vi "Drive straight.vi"(8 "Start Time":dbl, 9 "Length(seconds)":dbl, 10 "Desired angle":dbl) -> (0 "Complete or not":bool, 2 "X Power":dbl)   [LabVIEW 2020]
uses:
  Robot Global Data.vi
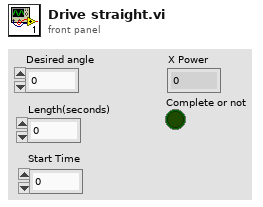
[diagram p1: front panel]
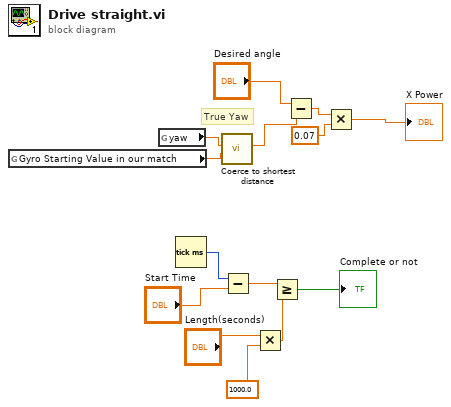
[diagram p0: block diagram]
diagram:
  # "True Yaw"
  n1 = global read "Robot Global Data.vi" "Gyro Starting Value in our match"() -> (w1:dbl)
  n2 = global read "Robot Global Data.vi" "yaw"() -> (w2:dbl)
  n3 = Tick Count (ms)() -> (millisecond timer value=w7:u32)
  n4 = call "Coerce to shortest distance.vi"("Angle 2"=w1, "Angle 1"=w2) -> ("Shortest distance"=w3:dbl)  [unwired: 9 in]
  n5 = Subtract(x=w7, y="Start Time") -> (x-y=w11:dbl)
  n6 = Multiply(x="Length(seconds)", y=1000.0) -> (x*y=w4:dbl)
  n7 = Greater Or Equal?(x=w11, y=w4) -> (x >= y?=→"Complete or not":bool)
  n8 = Subtract(x="Desired angle", y=w3) -> (x-y=w13:dbl)
  n9 = Multiply(x=w13, y=0.07) -> (x*y=→"X Power":dbl)
